vi "Connect by Direction.vi"(8 "error in (no error)":errorcluster, 9 "Direction":T1, 10 "From":T2, 11 "Maze in":refnum<class "Maze.lvclass">) -> (0 "error out":errorcluster, 1 "Out of Bounds":bool, 2 "Already Connected":bool, 3 "Maze out":refnum<class "Maze.lvclass">)   [LabVIEW 2020, in "Maze.lvlib" / "Maze.lvclass"]
uses:
  Maze.lvclass
  Position.ctl
  Direction.ctl
  Maze.lvclass/Maze.ctl
  Maze.lvlib
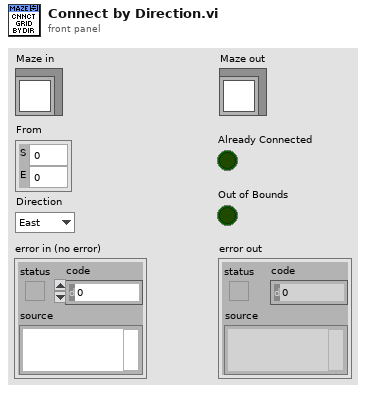
[diagram p1: front panel]
types:
  T1 = typedef "Maze.lvlib/Direction.ctl" = enum8{"East", "North", "West", "South"}
  T2 = typedef "Maze.lvlib/Position.ctl" = cluster{"S":i32, "E":i32}
  T3 = typedef "Maze.lvlib/Adjacency.ctl" = cluster{"E":bool, "N":bool, "W":bool, "S":bool, "Goal":bool, "Start":bool}
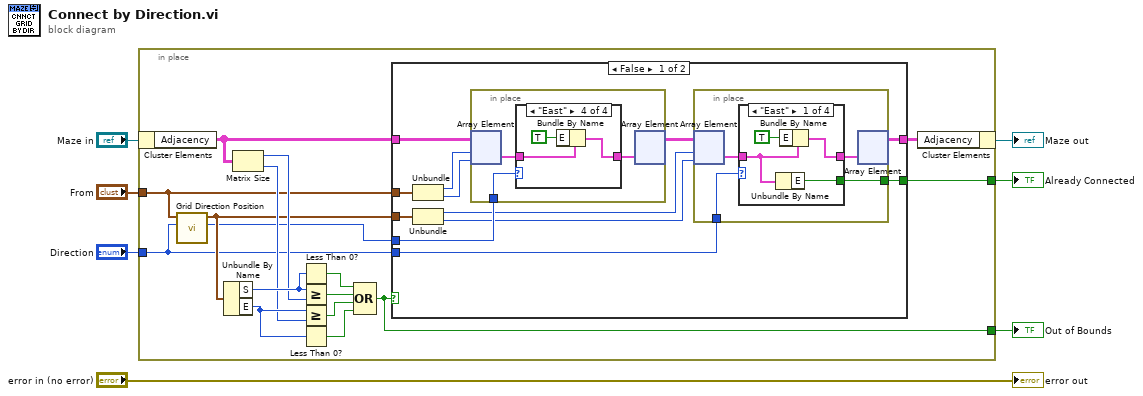
[diagram p0: block diagram]
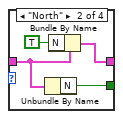
[diagram p2: hidden frame]
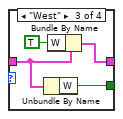
[diagram p3: hidden frame]
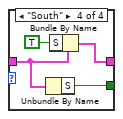
[diagram p4: hidden frame]
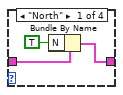
[diagram p5: hidden frame]
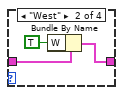
[diagram p6: hidden frame]
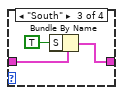
[diagram p7: hidden frame]
diagram:
  n1 = in-place {
    in-place-border: "From" -> [w12]
    in-place-border: "Direction" -> [w9]
    in-place-border: [w14] -> w3
    in-place-border: [w8] -> w1
    n2 = in-place-cluster #1("Maze in") -> ("Adjacency"=w15:T3[][])
    n3 = call "Grid Direction Position.vi"("Direction"=w9, "From"=w12) -> ("Opposite"=w10:T1, "To"=w11:T2)  [unwired: 8 in]
    n4 = Unbundle By Name(w11) -> ("S"=w23:i32, "E"=w21:i32)
    n5 = Matrix Size(0:w15) -> (1:w22:i32, 2:w20:i32)
    n6 = Less Than 0?(x=w23) -> (x < 0?=w16:bool)
    n7 = Greater Or Equal?(x=w23, y=w22) -> (x >= y?=w19:bool)
    n8 = Greater Or Equal?(x=w21, y=w20) -> (x >= y?=w18:bool)
    n9 = Less Than 0?(x=w21) -> (x < 0?=w17:bool)
    n10 = Compound Arithmetic op=OR(w16, w19, w18, w17) -> (w14:bool)
    n11 = case shown="False" w14 {
      tunnel: w15 -> [w33 w71]
      tunnel: [w25 w71] -> w13
      tunnel: w12 -> [w35 _]
      tunnel: w11 -> [w34 _]
      tunnel: w10 -> [w30 _]
      tunnel: w9 -> [w29 _]
      tunnel: [w24 _] -> w8
      frame False {
        n12 = Unbundle(w35) -> ("S"=w32:i32, "E"=w31:i32)
        n13 = Unbundle(w34) -> ("S"=w27:i32, "E"=w26:i32)
        n14 = in-place {
          in-place-border: w30 -> [w57]
          n15 = in-place-array #2(w33, w32, w31) -> (w58:T3)
          n16 = case shown="\"East\"" w57 {
            tunnel: w58 -> [w61 w64 w67 w70]
            tunnel: [w59 w62 w65 w68] -> w56
            frame "North" {
              n17 = Bundle By Name(cluster=w61, "N"=TRUE) -> (w59:T3)
            }
            frame "West" {
              n18 = Bundle By Name(cluster=w64, "W"=TRUE ("N")) -> (w62:T3)
            }
            frame "South" {
              n19 = Bundle By Name(cluster=w67, "S"=TRUE ("N")) -> (w65:T3)
            }
            frame "East" {
              n20 = Bundle By Name(cluster=w70, "E"=TRUE ("N")) -> (w68:T3)
            }
          }
          n21 = in-place-array #2(w56) -> (w28:T3[][])  [unwired: 2 out]
        }
        n22 = in-place {
          in-place-border: w29 -> [w38]
          in-place-border: [w36] -> w24
          n23 = in-place-array #3(w28, w27, w26) -> (w39:T3)
          n24 = case shown="\"East\"" w38 {
            tunnel: w39 -> [w41 w45 w49 w53]
            tunnel: [w42 w46 w50 w54] -> w37
            tunnel: [w40 w44 w48 w52] -> w36
            frame "East" {
              n25 = Unbundle By Name(w41) -> ("E"=w40:bool)
              n26 = Bundle By Name(cluster=w41, "E"=TRUE ("N")) -> (w42:T3)
            }
            frame "North" {
              n27 = Unbundle By Name(w45) -> ("N"=w44:bool)
              n28 = Bundle By Name(cluster=w45, "N"=TRUE) -> (w46:T3)
            }
            frame "West" {
              n29 = Unbundle By Name(w49) -> ("W"=w48:bool)
              n30 = Bundle By Name(cluster=w49, "W"=TRUE ("N")) -> (w50:T3)
            }
            frame "South" {
              n31 = Unbundle By Name(w53) -> ("S"=w52:bool)
              n32 = Bundle By Name(cluster=w53, "S"=TRUE ("N")) -> (w54:T3)
            }
          }
          n33 = in-place-array #3(w37) -> (w25:T3[][])  [unwired: 2 out]
        }
      }
      frame True {
      }
    }
    n34 = in-place-cluster #1("Adjacency"=w13) -> (→"Maze out":refnum<class "Maze.lvclass">)
  }
  "Already Connected" <- w1
  "Out of Bounds" <- w3
  "error out" <- "error in (no error)"
